vi "reward_behavior_michelle_visjitter_conswinAdapt_enticefx_TSLog_VF.vi"() -> ()   [LabVIEW 2019]
doc: "The myRIO Project template acquires acceleration data from the onboard accelerometer and displays the changes of acceleration values in a waveform chart."
uses:
  <vilib>/Analysis/Matrix/Datatypes/RealMatrix.ctl
  <vilib>/myRIO/Instrument Drivers/Onboard IO/DIO/typedefs/DIO Reference.ctl
  <vilib>/myRIO/Common/Instrument Driver Framework/Utilities/typedefs/myRIO Generic Hardware Reference.ctl
  <vilib>/myRIO/Common/Instrument Driver Framework/Utilities/typedefs/Hardware Version Enum.ctl
  <vilib>/myRIO/Common/Instrument Driver Framework/Utilities/typedefs/myRIO v1.0 Reference.ctl
  <vilib>/myRIO/Common/Instrument Driver Framework/Utilities/typedefs/Generic FPGA Reference.ctl
  <vilib>/myRIO/Common/Instrument Driver Framework/myRIO v1.0/DIO/typedefs/DIO Channels List.ctl
  <vilib>/myRIO/Common/Instrument Driver Framework/myRIO v1.0/DIO/typedefs/DIO Channels Enum.ctl
  <vilib>/userdefined/High Color/nirio_resource_hc.ctl
  <vilib>/myRIO/Common/Instrument Driver Framework/myRIO v1.0/Encoder/typedefs/Encoder Signal Mode.ctl
  <vilib>/myRIO/Instrument Drivers/Onboard IO/Encoder/typedefs/Encoder Reference.ctl
  <vilib>/myRIO/Common/Instrument Driver Framework/myRIO v1.0/Encoder/typedefs/Encoder Channels Enum.ctl
  <vilib>/myRIO/Common/Instrument Driver Framework/myRIO v1.0/Encoder/typedefs/Encoder Configuration v1.0.ctl
  <vilib>/myRIO/Common/Instrument Driver Framework/Utilities/vis/Is FPGA Ref Available.vi
  <vilib>/myRIO/Common/Instrument Driver Framework/myRIO v1.0/DIO/vis/myRIO v1.1 Open DIO.vi
  <vilib>/myRIO/Instrument Drivers/Onboard IO/DIO/vis/Write.vi
  <vilib>/myRIO/Common/Instrument Driver Framework/myRIO v1.0/Encoder/vis/myRIO v1.1 Open Encoder.vi
  <vilib>/myRIO/Instrument Drivers/Onboard IO/Encoder/vis/Read.vi
  <vilib>/myRIO/Instrument Drivers/Onboard IO/DIO/vis/Read.vi
  <vilib>/myRIO/Common/Instrument Driver Framework/Utilities/vis/Validate Channels.vi
  <vilib>/myRIO/Common/Instrument Driver Framework/myRIO v1.0/DIO/vis/myRIO v1.0 Reserve DIO.vi
  <vilib>/myRIO/Common/Instrument Driver Framework/myRIO v1.0/Encoder/vis/myRIO v1.0 Reserve Encoder.vi
  <vilib>/myRIO/Common/Instrument Driver Framework/myRIO v1.0/Resource Manager/vis/myRIO v1.0 Reserve Channel List.vi
  <vilib>/myRIO/Common/Instrument Driver Framework/myRIO v1.0/DIO/vis/myRIO v1.0 Build MUX Configuration DIO.vi
  <vilib>/myRIO/Common/Instrument Driver Framework/myRIO v1.0/Encoder/vis/myRIO v1.0 Build MUX Configuration Encoder.vi
  <vilib>/myRIO/Common/Instrument Driver Framework/myRIO v1.0/Resource Manager/vis/myRIO v1.0 Reserve Channel.vi
  <vilib>/myRIO/Common/Instrument Driver Framework/myRIO v1.0/Resource Manager/vis/myRIO v1.0 Unreserve Channel.vi
  <vilib>/myRIO/Common/Instrument Driver Framework/myRIO v1.0/Resource Manager/vis/myRIO v1.0 Create Configuration List.vi
  <vilib>/myRIO/Common/Instrument Driver Framework/myRIO v1.0/Resource Manager/vis/myRIO v1.0 Build Mutex Name.vi
  <vilib>/Utility/VariantDataType/GetNumericInfo.vi
  <vilib>/Utility/error.llb/Error Cluster From Error Code.vi
  <vilib>/myRIO/Common/Instrument Driver Framework/myRIO v1.0/myRIO v1.1 Open.vi
  <vilib>/myRIO/Common/Instrument Driver Framework/Utilities/vis/IO Manager.vi
  <vilib>/myRIO/Common/Instrument Driver Framework/Utilities/vis/Configuration Manager.vi
  <vilib>/myRIO/Common/Instrument Driver Framework/myRIO v1.0/Resource Manager/vis/myRIO v1.0 Configure IO.vi
  <vilib>/myRIO/Common/Instrument Driver Framework/myRIO v1.0/myRIO v1.0 Close.vi
  <vilib>/myRIO/Common/Instrument Driver Framework/myRIO v1.0/Encoder/vis/myRIO v1.0 Configure Encoder.vi
  <vilib>/myRIO/Common/Instrument Driver Framework/myRIO v1.0/Encoder/vis/myRIO v1.0 Read Encoder.vi
  <vilib>/myRIO/Common/Instrument Driver Framework/myRIO v1.0/DIO/vis/myRIO v1.0 Write DIO.vi
  <vilib>/myRIO/Common/Instrument Driver Framework/myRIO v1.0/DIO/vis/myRIO v1.0 Read DIO.vi
  <vilib>/myRIO/Express VI/Onboard IO/Encoder/Encoder Express VI.xnode
  <vilib>/myRIO/Instrument Drivers/Onboard IO/Encoder/vis/myRIO Encoder Open.xnode
  <vilib>/myRIO/Common/Instrument Driver Framework/myRIO v1.0/Encoder/typedefs/Encoder Count Direction Enum.ctl
  <vilib>/myRIO/Express VI/Onboard IO/DO/DO Express VI.xnode
  <vilib>/myRIO/Instrument Drivers/Onboard IO/DIO/vis/myRIO DIO Open.xnode
  <vilib>/myRIO/Express VI/Onboard IO/DI/DI Express VI.xnode
  <vilib>/myRIO/Instrument Drivers/Onboard IO/Encoder/Encoder.lvlib
  <vilib>/myRIO/Instrument Drivers/Onboard IO/DIO/DIO.lvlib
  <vilib>/Analysis/Matrix/NI_Matrix.lvlib
panel:
  out "AutoEnticeLimit":i32=1000
  out "GetVidFrame":i32
  out "VidTS":dbl[][](array[numeric])
  out "VidFrameClock":i32
  out "EntTS":dbl[][](array[numeric])
  out "TimeLag":dbl
  out "Lag2":dbl
  out "TestTime":dbl
  out "RewTS":dbl[][](array[numeric])
  out "ConsTS":dbl[][](array[numeric])
  out "LickTS":dbl[][](array[numeric])
  out "ContrastChoice":dbl
  out "Its":i32
  out "BurstCriteria":dbl
  out "LickBurst 2":bool
  out "LickBurst":bool
  out "Enticements":i32
  in  "Entice":bool
  out "Misses":i32
  out "GoAhead":bool
  out "TimeOutDuration":i32
  out "ActiveTime":dbl
  out "ConsumptionGo":bool=TRUE
  out "Consumption_Period":i32
  out "Watch_Display":bool=TRUE
  in  "Give reward":bool
  out "Timings":dbl[](array[numeric])
  out "ISI":dbl
  out "ISI start time":dbl
  out "Time_out":bool=TRUE
  out "Time since lick":dbl
  out "Time of last lick":dbl
  out "Rewarded trials":dbl[](array[numeric])
  out "Rewards":u16
  out "Active Trial":bool
  out "Array temp2":T1
  out "Stimuli Loaded":bool
  out "Stim_ID":dbl[](array[numeric])
  out "Reward_mat":dbl[](array[numeric])
  out "Reward":bool=TRUE
  out "Frame clock":i32
  out "Licks":u32
  out "Lick":bool
  out "Time":dbl
  out "Stop":bool
  in  "Frames to collect":u32
  out "Overflow?":bool
  out "Counter Value":i32
  out "Velocity":dbl
  out "Velocity Plot":dbl[](graph)
  out "Velocity array":dbl[](array[numeric])
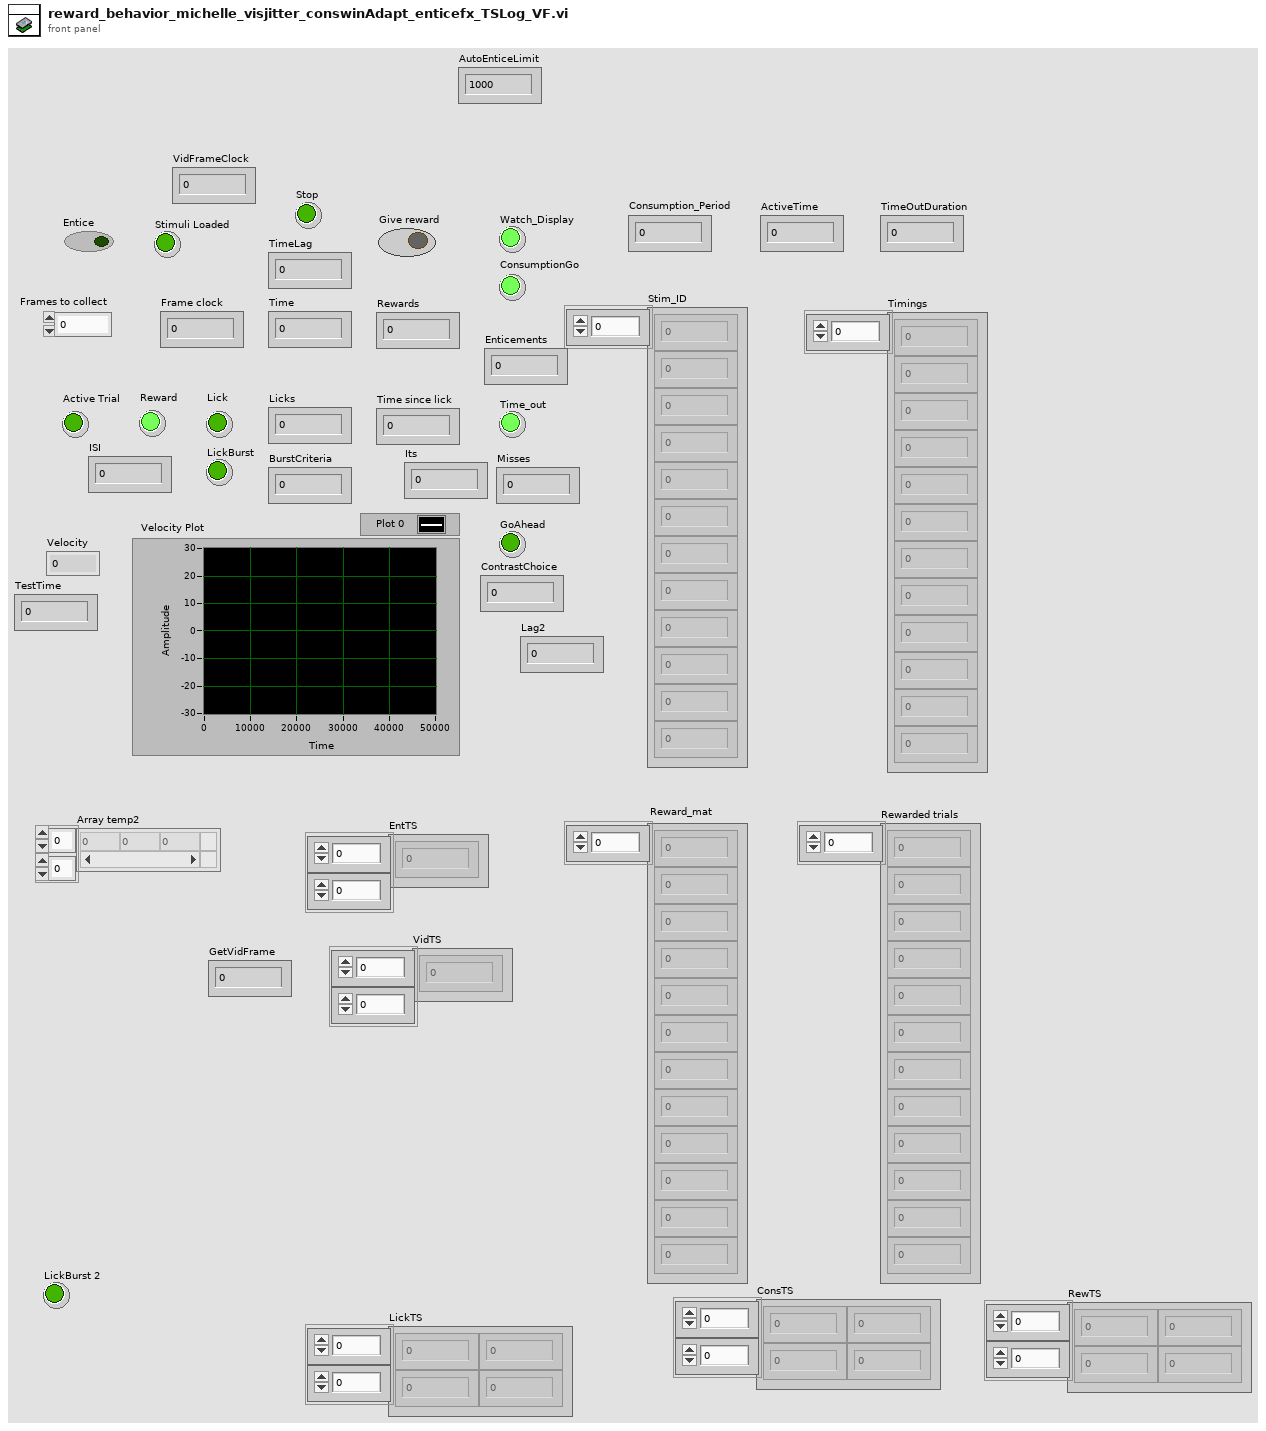
[diagram p1: front panel]
types:
  T1 = typedef "NI_Matrix.lvlib/RealMatrix.ctl" = dbl[][]
  T2 = typedef "DIO.lvlib/DIO Reference.ctl" = cluster{"myRIO Reference":T3, "DIO Channels List":T7}
  T3 = typedef "myRIO Generic Hardware Reference.ctl" = cluster{"myRIO Model":T4, "myRIO Hardware Reference":T5}
  T4 = typedef "Hardware Version Enum.ctl" = enum16{"Unknown", "myRIO-1900", "myRIO-1950", "roboRIO", "NI ELVIS RIO CM", "ELVIS III"}
  T5 = typedef "myRIO v1.0 Reference.ctl" = cluster{"Generic FPGA Reference":T6, "Allow multiple opens":bool}
  T6 = typedef "Generic FPGA Reference.ctl" = refnum<k20>
  T7 = typedef "DIO Channels List.ctl" = T8[]
  T8 = typedef "DIO Channels Enum.ctl" = enum16{"Not Connected", "C/DIO0", "C/DIO1", "C/DIO2", "C/DIO3", "C/DIO4", "C/DIO5", "C/DIO6", "C/DIO7", "A/DIO0", "A/DIO1", "A/DIO2", "A/DIO3", "A/DIO4", "A/DIO5", "A/DIO6", "A/DIO7", "A/DIO8", "A/DIO9", "A/DIO10", "A/DIO11", "A/DIO12", "A/DIO13", "A/DIO14", "A/DIO15", "A/DIO16", "A/DIO17", "A/DIO18", "A/DIO19", "B/DIO0", "B/DIO1", "B/DIO2", "B/DIO3", "B/DIO4", "B/DIO5", "B/DIO6", "B/DIO7", "B/DIO8", "B/DIO9", "B/DIO10", "B/DIO11", "B/DIO12", "B/DIO13", "B/DIO14", "B/DIO15", "B/DIO16", "B/DIO17", "B/DIO18", "B/DIO19", "LED0", "LED1", "LED2", "LED3", "Button0", "DIO/DIO0", "DIO/DIO1", "DIO/DIO2", "DIO/DIO3", "DIO/DIO4", "DIO/DIO5", "DIO/DIO6", "DIO/DIO7", "DIO/DIO8", "DIO/DIO9", "SPI/CS0", "SPI/CS1", "SPI/CS2", "SPI/CS3", "LED RADIO (Green)", "LED RADIO (Red)", "LED COMM (Green)", "LED COMM (Red)", "LED MODE (Green)", "LED MODE (Red)"}
  T9 = typedef "nirio_resource_hc.ctl" = tag
  T10 = typedef "Encoder.lvlib/Encoder Reference.ctl" = cluster{"myRIO Reference":T3, "Encoder Channels Enum":T11}
  T11 = typedef "Encoder Channels Enum.ctl" = enum16{"Not Connected", "C/ENC0", "C/ENC1", "A/ENC", "A/ENC0", "A/ENC1", "A/ENC2", "A/ENC3", "A/ENC4", "A/ENC5", "A/ENC6", "A/ENC7", "A/ENC8", "A/ENC9", "B/ENC", "B/ENC0", "B/ENC1", "B/ENC2", "B/ENC3", "B/ENC4", "B/ENC5", "B/ENC6", "B/ENC7", "B/ENC8", "B/ENC9", "DIO/ENC0", "DIO/ENC1", "DIO/ENC2", "DIO/ENC3", "DIO/ENC4"}
  T12 = typedef "Encoder Signal Mode.ctl" = enum16{"Quadrature phase signal", "Step and direction signal"}
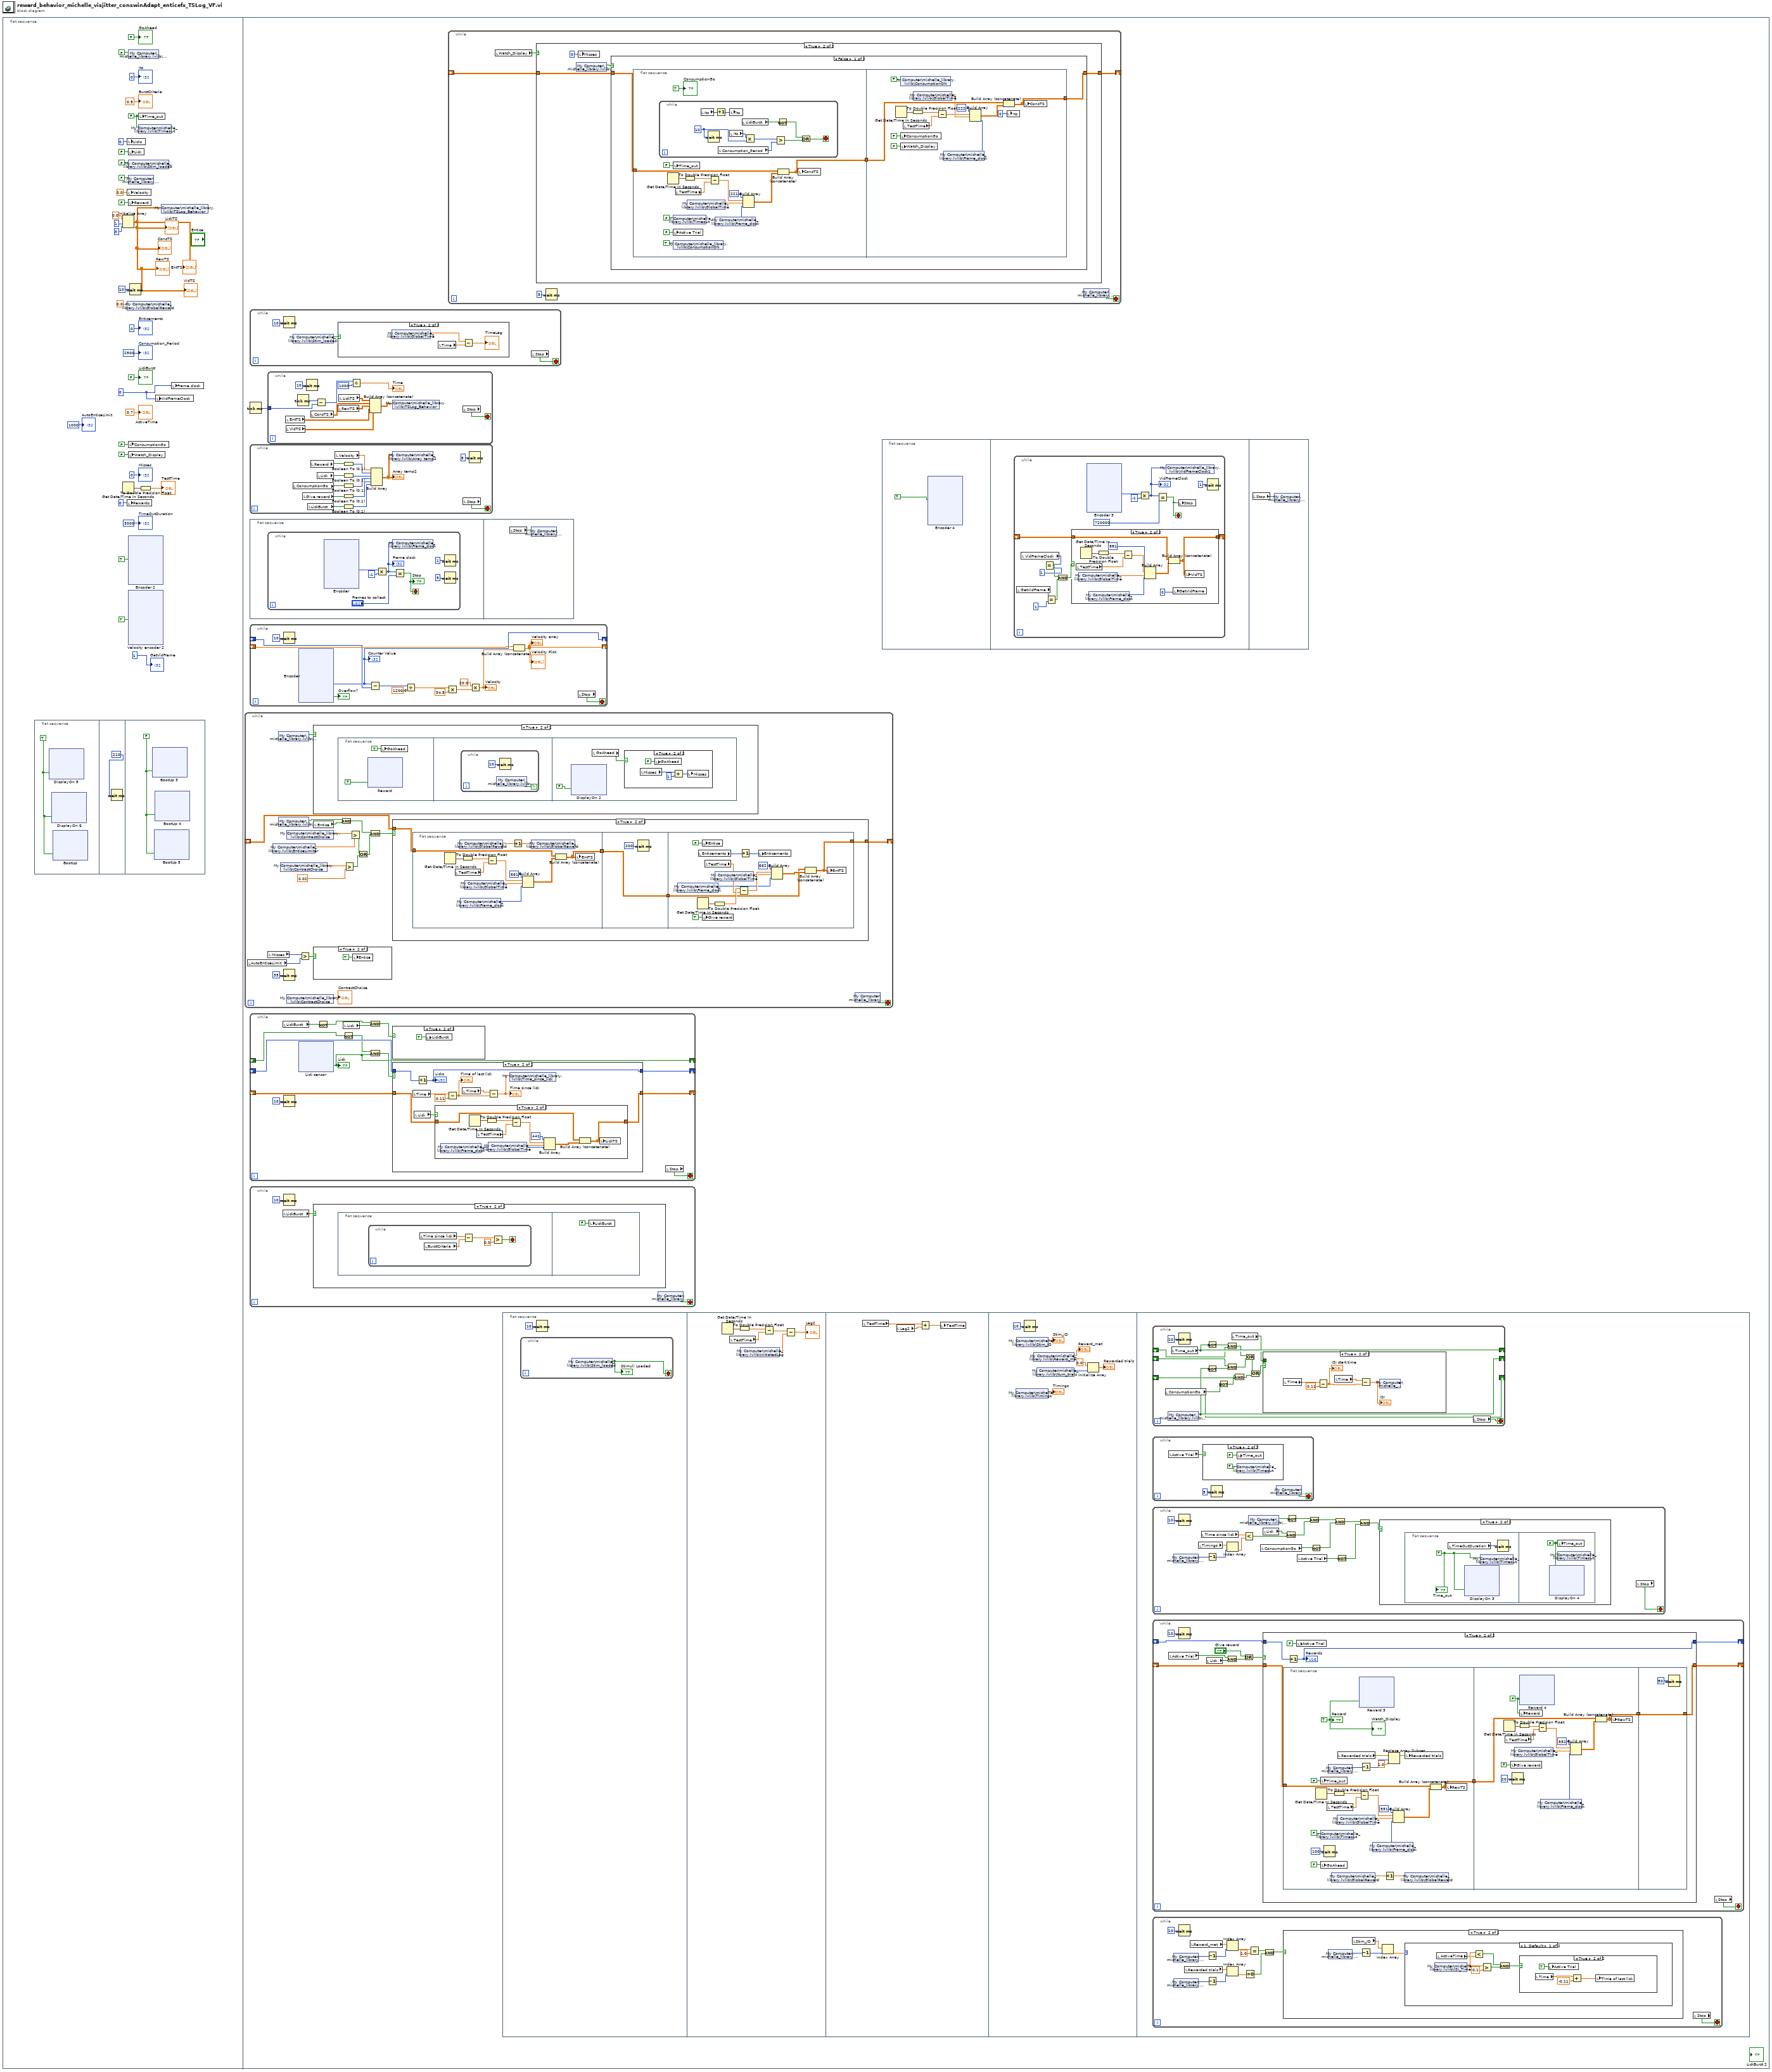
[diagram p0: block diagram]
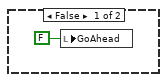
[diagram p7: hidden frame]
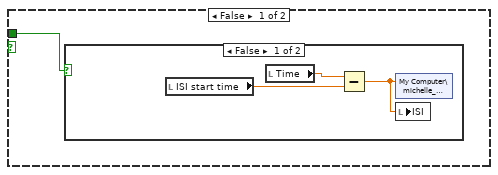
[diagram p13: hidden frame]
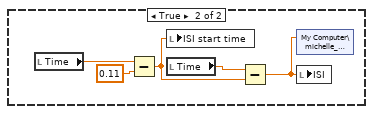
[diagram p14: hidden frame]
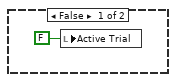
[diagram p15: hidden frame]
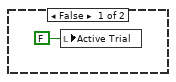
[diagram p16: hidden frame]
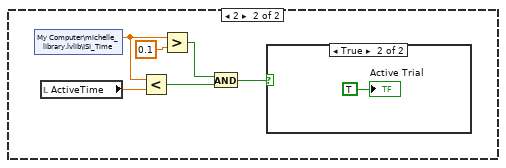
[diagram p17: hidden frame]
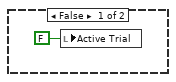
[diagram p18: hidden frame]
diagram:
  n1 = flat-sequence {
    frame #0 {
      w22 = FALSE ("Time_out")
      w4 = u32 0 ("Frames")
      n2 = flat-sequence {
        frame #0 {
          w34 = TRUE
          n3 = xnode "DisplayOn 5"("C/DIO2 (DIO2)"=w34) -> ()  [unwired: 1 in, 1 out]
          n4 = xnode "DisplayOn 6"("C/DIO1 (DIO1)"=w34) -> ()  [unwired: 1 in, 1 out]
          n5 = xnode "BootUp"("C/DIO3 (DIO3)"=w34) -> ()  [unwired: 1 in, 1 out]
        }
        frame #1 {
          n6 = Wait (ms)(milliseconds to wait=210) -> ()  [unwired: 1 out]
        }
        frame #2 {
          w141 = FALSE
          n7 = xnode "BootUp 3"("C/DIO2 (DIO2)"=w141) -> ()  [unwired: 1 in, 1 out]
          n8 = xnode "BootUp 5"("C/DIO3 (DIO3)"=w141) -> ()  [unwired: 1 in, 1 out]
          n9 = xnode "BootUp 4"("C/DIO1 (DIO1)"=w141) -> ()  [unwired: 1 in, 1 out]
        }
      }
      n10 = Get Date/Time In Seconds() -> (seconds since 1Jan1904=w6:timestamp)
      n11 = Initialize Array(0.0, 1, 3) -> (w3:dbl[][])
      "LickTS" <- w3
      "ConsTS" <- w3
      "RewTS" <- w3
      "EntTS" <- w3
      "VidTS" <- w3
      n12 = local write "Licks"(u32 0 ("Licks")) -> ()
      n13 = local write "Velocity"(0.0 ("Velocity")) -> ()
      n14 = shared-variable "My Computer\\michelle_library.lvlib\\GlobalReward"(0.0) -> ()  [unwired: 1 in, 1 out]
      n15 = local write "Rewards"(u16 0 ("Rewards")) -> ()
      n16 = shared-variable "My Computer\\michelle_library.lvlib\\Display"(FALSE ("Display")) -> ()  [unwired: 1 in, 1 out]
      n17 = local write "Lick"(FALSE ("Lick")) -> ()
      n18 = shared-variable "My Computer\\michelle_library.lvlib\\Stim_loaded"(FALSE ("Stim_loaded")) -> ()  [unwired: 1 in, 1 out]
      n19 = shared-variable "My Computer\\michelle_library.lvlib\\Stop"(FALSE ("Stop")) -> ()  [unwired: 1 in, 1 out]
      n20 = local write "Reward"(FALSE ("Give reward")) -> ()
      n21 = local write "ConsumptionGo"(FALSE ("ConsumptionGo")) -> ()
      n22 = local write "Watch_Display"(FALSE ("Watch_Display")) -> ()
      n23 = xnode "Encoder 2"("Reset Counter"=TRUE) -> ()  [unwired: 1 in, 4 out]
      n24 = xnode "Velocity encoder 2"("Reset Counter"=TRUE) -> ()  [unwired: 1 in, 4 out]
      n25 = Wait (ms)(milliseconds to wait=u32 10) -> ()  [unwired: 1 out]
      n26 = local write "Time_out"(w22) -> ()
      n27 = shared-variable "My Computer\\michelle_library.lvlib\\Timeout"(w22) -> ()  [unwired: 1 in, 1 out]
      n28 = To Double Precision Float(number=w6) -> (double precision float=→"TestTime":dbl)
      n29 = local write "VidFrameClock"(w4) -> ()
      n30 = shared-variable "My Computer\\michelle_library.lvlib\\TSLog_Behavior"(w3) -> ()  [unwired: 1 in, 1 out]
      n31 = local write "Frame clock"(w4) -> ()
      "Consumption_Period" <- 2500
      "ActiveTime" <- 0.7
      "TimeOutDuration" <- 3000
      "GoAhead" <- FALSE
      "Misses" <- 0
      "Enticements" <- 0
      "LickBurst" <- FALSE
      "BurstCriteria" <- 0.5
      "Its" <- 0
      "GetVidFrame" <- 1
      "AutoEnticeLimit" <- 1000
    }
    frame #1 {
      n32 = while {
        shift-right: [w484] -> _
        shift-left: _ -> [w485]
        stop <- w495 stop-if-true
        n33 = local read "AutoEnticeLimit"() -> (w476:i32)
        n34 = local read "Misses"() -> (w477:i32)
        n35 = shared-variable "My Computer\\michelle_library.lvlib\\EnticeLimiter"() -> (w483:dbl)  [unwired: 1 in, 1 out]
        n36 = shared-variable "My Computer\\michelle_library.lvlib\\Display"() -> (w494:bool)  [unwired: 1 in, 1 out]
        n37 = shared-variable "My Computer\\michelle_library.lvlib\\Display"() -> (w492:bool)  [unwired: 1 in, 1 out]
        n38 = shared-variable "My Computer\\michelle_library.lvlib\\ContrastChoice"() -> (w479:dbl)  [unwired: 1 in, 1 out]
        n39 = Wait (ms)(milliseconds to wait=35) -> ()  [unwired: 1 out]
        n40 = shared-variable "My Computer\\michelle_library.lvlib\\ContrastChoice"() -> (w488:dbl)  [unwired: 1 in, 1 out]
        n41 = shared-variable "My Computer\\michelle_library.lvlib\\ContrastChoice"() -> (→"ContrastChoice":dbl)  [unwired: 1 in, 1 out]
        n42 = Greater?(x=w477, y=w476) -> (0:w493:bool)
        n43 = case shown="True" w494 {
          frame False {
            n44 = local write "GoAhead"(FALSE) -> ()
          }
          frame True {
            n45 = flat-sequence {
              frame #0 {
                n46 = xnode "Reward"("C/DIO2 (DIO2)"=TRUE) -> ()  [unwired: 1 in, 1 out]
                n47 = local write "GoAhead"(TRUE) -> ()
              }
              frame #1 {
                n48 = while {
                  stop <- w569 continue-if-true
                  n49 = shared-variable "My Computer\\michelle_library.lvlib\\Display"() -> (w569:bool)  [unwired: 1 in, 1 out]
                  n50 = Wait (ms)(milliseconds to wait=10) -> ()  [unwired: 1 out]
                }
              }
              frame #2 {
                n51 = xnode "DisplayOn 2"("C/DIO2 (DIO2)"=FALSE) -> ()  [unwired: 1 in, 1 out]
                n52 = local read "GoAhead"() -> (w571:bool)
                n53 = case shown="True" w571 {
                  frame False {
                  }
                  frame True {
                    n54 = local read "Misses"() -> (w610:i32)
                    n55 = local write "GoAhead"(FALSE) -> ()
                    n56 = Add(x=w610, y=1) -> (x+y=w608:i32)
                    n57 = local write "Misses"(w608) -> ()
                  }
                }
              }
            }
          }
        }
        n58 = local read "Entice"() -> (w491:bool)
        n59 = case shown="True" w493 {
          frame False {
          }
          frame True {
            n60 = local write "Entice"(TRUE) -> ()
          }
        }
        n61 = And(x=w492, y=w491) -> (x .and. y?=w489:bool)
        n62 = Greater?(x=w479, y=0.02) -> (0:w480:bool)
        n63 = Greater?(x=w488, y=w483) -> (0:w481:bool)
        n64 = Or(x=w481, y=w480) -> (x .or. y?=w482:bool)
        n65 = And(x=w489, y=w482) -> (x .and. y?=w487:bool)
        n66 = case shown="True" w487 {
          tunnel: w485 -> [w496 w500]
          tunnel: [w496 w497] -> w484
          frame False {
          }
          frame True {
            n67 = flat-sequence {
              tunnel: w500 -> [w503]
              tunnel: [w502] -> w499
              tunnel: w499 -> [w513]
              tunnel: [w513] -> w498
              tunnel: w498 -> [w517]
              tunnel: [w516] -> w497
              frame #0 {
                n68 = Get Date/Time In Seconds() -> (seconds since 1Jan1904=w510:timestamp)
                n69 = local read "TestTime"() -> (w505:dbl)
                n70 = shared-variable "My Computer\\michelle_library.lvlib\\GlobalReward"() -> (w512:dbl)  [unwired: 1 in, 1 out]
                n71 = shared-variable "My Computer\\michelle_library.lvlib\\Frame_clock"() -> (w501:u32)  [unwired: 1 in, 1 out]
                n72 = To Double Precision Float(number=w510) -> (double precision float=w509:dbl)
                n73 = shared-variable "My Computer\\michelle_library.lvlib\\GlobalTime"() -> (w504:dbl)  [unwired: 1 in, 1 out]
                n74 = Subtract(x=w509, y=w505) -> (x-y=w508:dbl)
                n75 = Increment(x=w512) -> (x+1=w511:dbl)
                n76 = Build Array(661, w508, w504, w501) -> (w507:T1)
                n77 = shared-variable "My Computer\\michelle_library.lvlib\\GlobalReward"(w511) -> ()  [unwired: 1 in, 1 out]
                n78 = Build Array (concatenate) ("Build Matrix")(w503, w507) -> (w502:T1)
                n79 = local write "EntTS"(w502) -> ()
              }
              frame #1 {
                n80 = Wait (ms)(milliseconds to wait=200) -> ()  [unwired: 1 out]
              }
              frame #2 {
                n81 = shared-variable "My Computer\\michelle_library.lvlib\\Frame_clock"() -> (w515:u32)  [unwired: 1 in, 1 out]
                n82 = Get Date/Time In Seconds() -> (seconds since 1Jan1904=w524:timestamp)
                n83 = local read "Enticements"() -> (w526:i32)
                n84 = local write "Entice"(FALSE) -> ()
                n85 = local write "Give reward"(TRUE) -> ()
                n86 = local read "TestTime"() -> (w518:dbl)
                n87 = To Double Precision Float(number=w524) -> (double precision float=w523:dbl)
                n88 = shared-variable "My Computer\\michelle_library.lvlib\\GlobalTime"() -> (w519:dbl)  [unwired: 1 in, 1 out]
                n89 = Subtract(x=w523, y=w518) -> (x-y=w522:dbl)
                n90 = Increment(x=w526) -> (x+1=w525:i32)
                n91 = local write "Enticements"(w525) -> ()
                n92 = Build Array(662, w522, w519, w515) -> (w521:T1)
                n93 = Build Array (concatenate) ("Build Matrix")(w517, w521) -> (w516:T1)
                n94 = local write "EntTS"(w516) -> ()
              }
            }
          }
        }
        n95 = shared-variable "My Computer\\michelle_library.lvlib\\Stop"() -> (w495:bool)  [unwired: 1 in, 1 out]
      }
      n96 = while {
        stop <- w462 stop-if-true
        n97 = Wait (ms)(milliseconds to wait=u32 10) -> ()  [unwired: 1 out]
        n98 = shared-variable "My Computer\\michelle_library.lvlib\\Stim_loaded"() -> (w463:bool)  [unwired: 1 in, 1 out]
        n99 = case shown="True" w463 {
          frame False {
          }
          frame True {
            n100 = shared-variable "My Computer\\michelle_library.lvlib\\GlobalTime"() -> (w464:dbl)  [unwired: 1 in, 1 out]
            n101 = local read "Time"() -> (w465:dbl)
            n102 = Subtract(x=w464, y=w465) -> (x-y=→"TimeLag":dbl)
          }
        }
        n103 = local read "Stop"() -> (w462:bool)
      }
      n104 = Tick Count (ms)() -> (millisecond timer value=w339:u32)
      n105 = while {
        stop <- w671 stop-if-true
        n106 = local read "ConsumptionGo"() -> (w669:bool)
        n107 = local read "Give reward"() -> (w668:bool)
        n108 = local read "LickBurst"() -> (w665:bool)
        n109 = local read "Reward"() -> (w676:bool)
        n110 = local read "Lick"() -> (w677:bool)
        n111 = local read "Velocity"() -> (w675:dbl)
        n112 = Boolean To (0,1)(Boolean=w676) -> (0, 1=w674:i16)
        n113 = Boolean To (0,1)(Boolean=w677) -> (0, 1=w673:i16)
        n114 = Boolean To (0,1)(Boolean=w669) -> (0, 1=w667:i16)
        n115 = Boolean To (0,1)(Boolean=w668) -> (0, 1=w666:i16)
        n116 = Boolean To (0,1)(Boolean=w665) -> (0, 1=w664:i16)
        n117 = Build Array(w675, w674, w673, w667, w666, w664) -> (w670:T1)
        "Array temp2" <- w670
        n118 = shared-variable "My Computer\\michelle_library.lvlib\\Array temp2"(w670) -> ()  [unwired: 1 in, 1 out]
        n119 = local read "Stop"() -> (w671:bool)
        n120 = Wait (ms)(milliseconds to wait=u32 5) -> ()  [unwired: 1 out]
      }
      n121 = flat-sequence {
        frame #0 {
          n122 = while {
            stop <- w990 stop-if-true
            n123 = xnode "Encoder"() -> ("Counter Value"=w994:i32)  [unwired: 2 in, 3 out]
            n124 = Multiply(x=w994, y=-1) -> (x*y=w989:i32)
            "Frame clock" <- w989
            n125 = shared-variable "My Computer\\michelle_library.lvlib\\Frame_clock"(w989) -> ()  [unwired: 1 in, 1 out]
            n126 = Equal?(x=w989, y="Frames to collect") -> (x = y?=w990:bool)
            "Stop" <- w990
            n127 = Wait (ms)(milliseconds to wait=u32 1) -> ()  [unwired: 1 out]
            n128 = Wait (ms)(milliseconds to wait=u32 5) -> ()  [unwired: 1 out]
          }
        }
        frame #1 {
          n129 = local read "Stop"() -> (w1042:bool)
          n130 = shared-variable "My Computer\\michelle_library.lvlib\\Stop"(w1042) -> ()  [unwired: 1 in, 1 out]
        }
      }
      n131 = while {
        shift-right: [w1129] -> _
        shift-left: _ -> [w1130]
        shift-right: [w1121] -> _
        shift-left: _ -> [w1120]
        stop <- w1119 stop-if-true
        n132 = Wait (ms)(milliseconds to wait=u32 10) -> ()  [unwired: 1 out]
        n133 = xnode "Encoder"() -> ("Counter Value"=w1129:i32, "Overflow?"=→"Overflow?":bool)  [unwired: 2 in, 2 out]
        "Counter Value" <- w1129
        n134 = Subtract(x=w1129, y=w1130) -> (x-y=w1122:i32)
        n135 = Divide(x=w1122, y=1200.0 ("600")) -> (x/y=w1127:dbl)
        n136 = Multiply(x=w1127, y=34.5) -> (x*y=w1125:dbl)
        n137 = Multiply(x=20.0, y=w1125) -> (x*y=w1123:dbl)
        "Velocity" <- w1123
        n138 = Build Array (concatenate)(w1120, w1123) -> (w1121:dbl[])
        "Velocity Plot" <- w1121
        "Velocity array" <- w1121
        n139 = local read "Stop"() -> (w1119:bool)
      }
      n140 = while {
        shift-right: [w1055] -> _
        shift-left: _ -> [w1054]
        shift-right: [w1049] -> _
        shift-left: _ -> [w1052]
        shift-right: [w1043] -> _
        shift-left: _ -> [w1044]
        stop <- w1053 stop-if-true
        n141 = local read "LickBurst"() -> (w1046:bool)
        n142 = Wait (ms)(milliseconds to wait=u32 10) -> ()  [unwired: 1 out]
        n143 = xnode "Lick sensor"() -> ("C/DIO1 (DIO1)"=w1049:bool)  [unwired: 1 in, 1 out]
        "Lick" <- w1049
        n144 = Not(x=w1046) -> (.not. x?=w1045:bool)
        n145 = Not(x=w1052) -> (.not. x?=w1051:bool)
        n146 = local read "Lick"() -> (w1047:bool)
        n147 = And(x=w1045, y=w1047) -> (x .and. y?=w1048:bool)
        n148 = And(x=w1051, y=w1049) -> (x .and. y?=w1050:bool)
        n149 = case shown="True" w1048 {
          frame False {
          }
          frame True {
            n150 = local write "LickBurst"(TRUE) -> ()
          }
        }
        n151 = case shown="True" w1050 {
          tunnel: [w1062 w1072] -> w1055
          tunnel: w1054 -> [w1062 w1071]
          tunnel: w1044 -> [w1058 w1063]
          tunnel: [w1058 w1065] -> w1043
          frame False {
            n152 = local read "Time of last lick"() -> (w1060:dbl)
            n153 = local read "Time"() -> (w1061:dbl)
            n154 = Subtract(x=w1061, y=w1060) -> (x-y=w1059:dbl)
            n155 = shared-variable "My Computer\\michelle_library.lvlib\\Time_since_lick"(w1059) -> ()  [unwired: 1 in, 1 out]
            n156 = local write "Time since lick"(w1059) -> ()
          }
          frame True {
            n157 = local read "Time"() -> (w1068:dbl)
            n158 = local read "Lick"() -> (w1064:bool)
            n159 = Increment(x=w1071) -> (x+1=w1072:u32)
            "Licks" <- w1072
            n160 = case shown="True" w1064 {
              tunnel: w1063 -> [w1073 w1079]
              tunnel: [w1073 w1078] -> w1065
              frame False {
              }
              frame True {
                n161 = shared-variable "My Computer\\michelle_library.lvlib\\Frame_clock"() -> (w1074:u32)  [unwired: 1 in, 1 out]
                n162 = Get Date/Time In Seconds() -> (seconds since 1Jan1904=w1081:timestamp)
                n163 = local read "TestTime"() -> (w1076:dbl)
                n164 = To Double Precision Float(number=w1081) -> (double precision float=w1077:dbl)
                n165 = shared-variable "My Computer\\michelle_library.lvlib\\GlobalTime"() -> (w1075:dbl)  [unwired: 1 in, 1 out]
                n166 = Subtract(x=w1077, y=w1076) -> (x-y=w1082:dbl)
                n167 = Build Array(441, w1082, w1075, w1074) -> (w1083:T1)
                n168 = Build Array (concatenate) ("Build Matrix")(w1079, w1083) -> (w1078:T1)
                n169 = local write "LickTS"(w1078) -> ()
              }
            }
            n170 = Subtract(x=w1068, y=0.11) -> (x-y=w1066:dbl)
            "Time of last lick" <- w1066
            n171 = local read "Time"() -> (w1070:dbl)
            n172 = Subtract(x=w1070, y=w1066) -> (x-y=w1069:dbl)
            "Time since lick" <- w1069
            n173 = shared-variable "My Computer\\michelle_library.lvlib\\Time_since_lick"(w1069) -> ()  [unwired: 1 in, 1 out]
          }
        }
        n174 = local read "Stop"() -> (w1053:bool)
      }
      n175 = while {
        stop <- w469 stop-if-true
        n176 = local read "LickBurst"() -> (w467:bool)
        n177 = Wait (ms)(milliseconds to wait=u32 10) -> ()  [unwired: 1 out]
        n178 = case shown="True" w467 {
          frame False {
          }
          frame True {
            n179 = flat-sequence {
              frame #0 {
                n180 = while {
                  stop <- w472 stop-if-true
                  n181 = local read "Time since lick"() -> (w473:dbl)
                  n182 = local read "BurstCriteria"() -> (w474:dbl)
                  n183 = Subtract(x=w473, y=w474) -> (x-y=w470:dbl)
                  n184 = Greater?(x=w470, y=0.0) -> (0:w472:bool)
                }
              }
              frame #1 {
                n185 = local write "LickBurst"(FALSE) -> ()
              }
            }
          }
        }
        n186 = shared-variable "My Computer\\michelle_library.lvlib\\Stop"() -> (w469:bool)  [unwired: 1 in, 1 out]
      }
      n187 = while {
        tunnel: w339 -> [w1190]
        stop <- w1188 stop-if-true
        n188 = local read "EntTS"() -> (w1180:dbl[][])
        n189 = local read "VidTS"() -> (w1179:dbl[][])
        n190 = Tick Count (ms)() -> (millisecond timer value=w1191:u32)
        n191 = Wait (ms)(milliseconds to wait=u32 10) -> ()  [unwired: 1 out]
        n192 = local read "ConsTS"() -> (w1183:dbl[][])
        n193 = Subtract(x=w1191, y=w1190) -> (x-y=w1187:u32)
        n194 = local read "RewTS"() -> (w1182:dbl[][])
        n195 = local read "LickTS"() -> (w1184:dbl[][])
        n196 = Divide(x=w1187, y=u32 1000) -> (x/y=→"Time":dbl)
        n197 = Build Array (concatenate) ("Build Matrix")(w1184, w1183, w1182, w1180, w1179) -> (w1181:T1)
        n198 = shared-variable "My Computer\\michelle_library.lvlib\\TSLog_Behavior"(w1181) -> ()  [unwired: 1 in, 1 out]
        n199 = local read "Stop"() -> (w1188:bool)
      }
      n200 = while {
        shift-right: [w611] -> _
        shift-left: _ -> [w612]
        stop <- w615 stop-if-true
        n201 = local read "Watch_Display"() -> (w614:bool)
        n202 = case shown="True" w614 {
          tunnel: w612 -> [w616 w618]
          tunnel: [w616 w617] -> w611
          frame False {
          }
          frame True {
            n203 = shared-variable "My Computer\\michelle_library.lvlib\\Display"() -> (w620:bool)  [unwired: 1 in, 1 out]
            n204 = local write "Misses"(0) -> ()
            n205 = case shown="False" w620 {
              tunnel: w618 -> [w623 w663]
              tunnel: [w621 w663] -> w617
              frame False {
                n206 = flat-sequence {
                  tunnel: w623 -> [w627]
                  tunnel: [w626] -> w622
                  tunnel: w622 -> [w653]
                  tunnel: [w652] -> w621
                  frame #0 {
                    n207 = while {
                      stop <- w642 stop-if-true
                      w643 = 10
                      n208 = local read "Its"() -> (w647:i32)
                      n209 = Wait (ms)(milliseconds to wait=w643) -> ()  [unwired: 1 out]
                      n210 = Increment(x=w647) -> (x+1=w646:i32)
                      n211 = local read "Consumption_Period"() -> (w640:i32)
                      n212 = local write "Its"(w646) -> ()
                      n213 = local read "Its"() -> (w644:i32)
                      n214 = local read "LickBurst"() -> (w648:bool)
                      n215 = Multiply(x=w644, y=w643) -> (x*y=w641:i32)
                      n216 = Greater?(x=w641, y=w640) -> (0:w639:bool)
                      n217 = Not(x=w648) -> (.not. x?=w645:bool)
                      n218 = Or(x=w645, y=w639) -> (x .or. y?=w642:bool)
                    }
                    n219 = Get Date/Time In Seconds() -> (seconds since 1Jan1904=w632:timestamp)
                    n220 = local write "Time_out"(FALSE) -> ()
                    n221 = shared-variable "My Computer\\michelle_library.lvlib\\Timeout"(FALSE) -> ()  [unwired: 1 in, 1 out]
                    n222 = local write "Active Trial"(FALSE) -> ()
                    n223 = shared-variable "My Computer\\michelle_library.lvlib\\ConsumptionON"(TRUE) -> ()  [unwired: 1 in, 1 out]
                    n224 = local read "TestTime"() -> (w629:dbl)
                    n225 = To Double Precision Float(number=w632) -> (double precision float=w630:dbl)
                    n226 = shared-variable "My Computer\\michelle_library.lvlib\\GlobalTime"() -> (w625:dbl)  [unwired: 1 in, 1 out]
                    n227 = Subtract(x=w630, y=w629) -> (x-y=w633:dbl)
                    n228 = shared-variable "My Computer\\michelle_library.lvlib\\Frame_clock"() -> (w624:u32)  [unwired: 1 in, 1 out]
                    n229 = Build Array(221, w633, w625, w624) -> (w628:T1)
                    n230 = Build Array (concatenate) ("Build Matrix")(w627, w628) -> (w626:T1)
                    n231 = local write "ConsTS"(w626) -> ()
                    "ConsumptionGo" <- TRUE
                  }
                  frame #1 {
                    n232 = Get Date/Time In Seconds() -> (seconds since 1Jan1904=w657:timestamp)
                    n233 = shared-variable "My Computer\\michelle_library.lvlib\\ConsumptionON"(FALSE) -> ()  [unwired: 1 in, 1 out]
                    n234 = local write "ConsumptionGo"(FALSE ("ConsumptionGo")) -> ()
                    n235 = local write "Watch_Display"(FALSE ("Watch_Display")) -> ()
                    n236 = local read "TestTime"() -> (w654:dbl)
                    n237 = To Double Precision Float(number=w657) -> (double precision float=w655:dbl)
                    n238 = shared-variable "My Computer\\michelle_library.lvlib\\GlobalTime"() -> (w650:dbl)  [unwired: 1 in, 1 out]
                    n239 = Subtract(x=w655, y=w654) -> (x-y=w658:dbl)
                    n240 = shared-variable "My Computer\\michelle_library.lvlib\\Frame_clock"() -> (w649:u32)  [unwired: 1 in, 1 out]
                    n241 = Build Array(222, w658, w650, w649) -> (w651:T1)
                    n242 = Build Array (concatenate) ("Build Matrix")(w653, w651) -> (w652:T1)
                    n243 = local write "Its"(0) -> ()
                    n244 = local write "ConsTS"(w652) -> ()
                  }
                }
              }
              frame True {
              }
            }
          }
        }
        n245 = Wait (ms)(milliseconds to wait=u32 5) -> ()  [unwired: 1 out]
        n246 = shared-variable "My Computer\\michelle_library.lvlib\\Stop"() -> (w615:bool)  [unwired: 1 in, 1 out]
      }
      n247 = flat-sequence {
        frame #0 {
          n248 = while {
            stop <- w679 stop-if-true
            n249 = shared-variable "My Computer\\michelle_library.lvlib\\Stim_loaded"() -> (w679:bool)  [unwired: 1 in, 1 out]
            "Stimuli Loaded" <- w679
          }
          n250 = Wait (ms)(milliseconds to wait=u32 10) -> ()  [unwired: 1 out]
        }
        frame #1 {
          n251 = Get Date/Time In Seconds() -> (seconds since 1Jan1904=w685:timestamp)
          n252 = local read "TestTime"() -> (w684:dbl)
          n253 = To Double Precision Float(number=w685) -> (double precision float=w683:dbl)
          n254 = shared-variable "My Computer\\michelle_library.lvlib\\InitiatedLag"() -> (w682:dbl)  [unwired: 1 in, 1 out]
          n255 = Subtract(x=w683, y=w684) -> (x-y=w680:dbl)
          n256 = Subtract(x=w680, y=w682) -> (x-y=→"Lag2":dbl)
        }
        frame #2 {
          n257 = local read "TestTime"() -> (w686:dbl)
          n258 = local read "Lag2"() -> (w687:dbl)
          n259 = Add(x=w686, y=w687) -> (x+y=w688:dbl)
          n260 = local write "TestTime"(w688) -> ()
        }
        frame #3 {
          n261 = shared-variable "My Computer\\michelle_library.lvlib\\Timings"() -> (→"Timings":dbl[])  [unwired: 1 in, 1 out]
          n262 = shared-variable "My Computer\\michelle_library.lvlib\\Stim_ID"() -> (→"Stim_ID":dbl[])  [unwired: 1 in, 1 out]
          n263 = Wait (ms)(milliseconds to wait=u32 10) -> ()  [unwired: 1 out]
          n264 = shared-variable "My Computer\\michelle_library.lvlib\\Reward_mat"() -> (→"Reward_mat":dbl[])  [unwired: 1 in, 1 out]
          n265 = shared-variable "My Computer\\michelle_library.lvlib\\Num_trials"() -> (w692:u32)  [unwired: 1 in, 1 out]
          n266 = Initialize Array(0.0 ("element"), w692) -> (→"Rewarded trials":dbl[])
        }
        frame #4 {
          n267 = while {
            shift-right: [w808] -> _
            shift-left: _ -> [w806]
            shift-right: [w804] -> _
            shift-left: _ -> [w803]
            shift-right: [w798] -> _
            shift-left: _ -> [w796]
            stop <- w809 stop-if-true
            n268 = local read "ConsumptionGo"() -> (w798:bool)
            n269 = shared-variable "My Computer\\michelle_library.lvlib\\Display"() -> (w804:bool)  [unwired: 1 in, 1 out]
            n270 = local read "Time_out"() -> (w808:bool)
            n271 = Wait (ms)(milliseconds to wait=u32 10) -> ()  [unwired: 1 out]
            n272 = Not(x=w808) -> (.not. x?=w807:bool)
            n273 = Not(x=w804) -> (.not. x?=w802:bool)
            n274 = Not(x=w798) -> (.not. x?=w799:bool)
            n275 = And(x=w807, y=w806) -> (x .and. y?=w801:bool)
            n276 = And(x=w803, y=w802) -> (x .and. y?=w797:bool)
            n277 = local read "Time_out"() -> (w805:bool)
            n278 = And(x=w796, y=w799) -> (x .and. y?=w795:bool)
            n279 = Or(x=w801, y=w797) -> (x .or. y?=w794:bool)
            n280 = Or(x=w794, y=w795) -> (x .or. y?=w793:bool)
            n281 = case shown="True" w793 {
              tunnel: w805 -> [w810 _]
              frame False {
                n282 = case shown="False" w810 {
                  frame False {
                    n283 = local read "ISI start time"() -> (w813:dbl)
                    n284 = local read "Time"() -> (w812:dbl)
                    n285 = Subtract(x=w812, y=w813) -> (x-y=w811:dbl)
                    n286 = shared-variable "My Computer\\michelle_library.lvlib\\ISI"(w811) -> ()  [unwired: 1 in, 1 out]
                    n287 = local write "ISI"(w811) -> ()
                  }
                  frame True {
                    n288 = local read "Time"() -> (w818:dbl)
                    n289 = Subtract(x=w818, y=0.11) -> (x-y=w815:dbl)
                    n290 = local write "ISI start time"(w815) -> ()
                    n291 = local read "Time"() -> (w816:dbl)
                    n292 = Subtract(x=w816, y=w815) -> (x-y=w814:dbl)
                    n293 = shared-variable "My Computer\\michelle_library.lvlib\\ISI"(w814) -> ()  [unwired: 1 in, 1 out]
                    n294 = local write "ISI"(w814) -> ()
                  }
                }
              }
              frame True {
                n295 = local read "Time"() -> (w823:dbl)
                n296 = Subtract(x=w823, y=0.11) -> (x-y=w820:dbl)
                "ISI start time" <- w820
                n297 = local read "Time"() -> (w821:dbl)
                n298 = Subtract(x=w821, y=w820) -> (x-y=w819:dbl)
                "ISI" <- w819
                n299 = shared-variable "My Computer\\michelle_library.lvlib\\ISI"(w819) -> ()  [unwired: 1 in, 1 out]
              }
            }
            n300 = local read "Stop"() -> (w809:bool)
          }
          n301 = while {
            stop <- w698 stop-if-true
            n302 = local read "Active Trial"() -> (w697:bool)
            n303 = case shown="True" w697 {
              frame False {
              }
              frame True {
                n304 = local write "Time_out"(FALSE) -> ()
                n305 = shared-variable "My Computer\\michelle_library.lvlib\\Timeout"(FALSE) -> ()  [unwired: 1 in, 1 out]
              }
            }
            n306 = Wait (ms)(milliseconds to wait=5) -> ()  [unwired: 1 out]
            n307 = shared-variable "My Computer\\michelle_library.lvlib\\Stop"() -> (w698:bool)  [unwired: 1 in, 1 out]
          }
          n308 = while {
            stop <- w719 stop-if-true
            n309 = shared-variable "My Computer\\michelle_library.lvlib\\Trial"() -> (w709:u32)  [unwired: 1 in, 1 out]
            n310 = Wait (ms)(milliseconds to wait=u32 10) -> ()  [unwired: 1 out]
            n311 = local read "Timings"() -> (w711:dbl[])
            n312 = local read "Time since lick"() -> (w718:dbl)
            n313 = Decrement(x=w709) -> (x-1=w708:u32)
            n314 = Index Array(array=w711, index=w708) -> (element=w710:dbl)
            n315 = Less?(x=w718, y=w710) -> (x < y?=w717:bool)
            n316 = shared-variable "My Computer\\michelle_library.lvlib\\Display"() -> (w714:bool)  [unwired: 1 in, 1 out]
            n317 = local read "ConsumptionGo"() -> (w706:bool)
            n318 = local read "Lick"() -> (w716:bool)
            n319 = And(x=w716, y=w717) -> (x .and. y?=w712:bool)
            n320 = Not(x=w714) -> (.not. x?=w713:bool)
            n321 = local read "Active Trial"() -> (w701:bool)
            n322 = And(x=w713, y=w712) -> (x .and. y?=w705:bool)
            n323 = Not(x=w706) -> (.not. x?=w707:bool)
            n324 = And(x=w705, y=w707) -> (x .and. y?=w703:bool)
            n325 = Not(x=w701) -> (.not. x?=w704:bool)
            n326 = And(x=w703, y=w704) -> (x .and. y?=w702:bool)
            n327 = case shown="True" w702 {
              frame False {
              }
              frame True {
                n328 = flat-sequence {
                  frame #0 {
                    w720 = TRUE
                    n329 = local read "TimeOutDuration"() -> (w721:i32)
                    n330 = xnode "DisplayOn 3"("C/DIO3 (DIO3)"=w720) -> ()  [unwired: 1 in, 1 out]
                    n331 = shared-variable "My Computer\\michelle_library.lvlib\\Timeout"(w720) -> ()  [unwired: 1 in, 1 out]
                    n332 = Wait (ms)(milliseconds to wait=w721) -> ()  [unwired: 1 out]
                    "Time_out" <- w720
                  }
                  frame #1 {
                    w757 = FALSE ("Timeout")
                    n333 = xnode "DisplayOn 4"("C/DIO3 (DIO3)"=w757) -> ()  [unwired: 1 in, 1 out]
                    n334 = local write "Time_out"(w757) -> ()
                    n335 = shared-variable "My Computer\\michelle_library.lvlib\\Timeout"(w757) -> ()  [unwired: 1 in, 1 out]
                  }
                }
              }
            }
            n336 = local read "Stop"() -> (w719:bool)
          }
          n337 = while {
            shift-right: [w870] -> _
            shift-left: _ -> [w869]
            shift-right: [w862] -> _
            shift-left: _ -> [w863]
            stop <- w872 stop-if-true
            n338 = local read "Active Trial"() -> (w867:bool)
            n339 = Wait (ms)(milliseconds to wait=u32 10) -> ()  [unwired: 1 out]
            n340 = local read "Lick"() -> (w868:bool)
            n341 = And(x=w867, y=w868) -> (x .and. y?=w866:bool)
            n342 = Or(x="Give reward", y=w866) -> (x .or. y?=w865:bool)
            n343 = case shown="True" w865 {
              tunnel: [w874 w881] -> w870
              tunnel: w869 -> [w874 w880]
              tunnel: w863 -> [w873 w878]
              tunnel: [w873 w877] -> w862
              frame False {
              }
              frame True {
                n344 = flat-sequence {
                  tunnel: w878 -> [w887]
                  tunnel: [w884] -> w875
                  tunnel: [w943] -> w876
                  tunnel: w875 -> [w941]
                  tunnel: [w987] -> w877
                  tunnel: w876 -> [w987]
                  frame #0 {
                    w902 = TRUE ("C/DIO0 (DIO0)")
                    n345 = Get Date/Time In Seconds() -> (seconds since 1Jan1904=w891:timestamp)
                    n346 = local write "Time_out"(FALSE) -> ()
                    n347 = shared-variable "My Computer\\michelle_library.lvlib\\Timeout"(FALSE) -> ()  [unwired: 1 in, 1 out]
                    n348 = local write "GoAhead"(FALSE) -> ()
                    n349 = Wait (ms)(milliseconds to wait=u32 100) -> ()  [unwired: 1 out]
                    n350 = local read "TestTime"() -> (w885:dbl)
                    n351 = shared-variable "My Computer\\michelle_library.lvlib\\Trial"() -> (w901:u32)  [unwired: 1 in, 1 out]
                    n352 = shared-variable "My Computer\\michelle_library.lvlib\\GlobalReward"() -> (w893:dbl)  [unwired: 1 in, 1 out]
                    n353 = To Double Precision Float(number=w891) -> (double precision float=w890:dbl)
                    n354 = shared-variable "My Computer\\michelle_library.lvlib\\GlobalTime"() -> (w883:dbl)  [unwired: 1 in, 1 out]
                    n355 = local read "Rewarded trials"() -> (w899:dbl[])
                    n356 = Subtract(x=w890, y=w885) -> (x-y=w889:dbl)
                    n357 = xnode "Reward 3"("C/DIO0 (DIO0)"=w902) -> ()  [unwired: 1 in, 1 out]
                    n358 = Decrement(x=w901) -> (x-1=w900:u32)
                    n359 = shared-variable "My Computer\\michelle_library.lvlib\\Frame_clock"() -> (w882:u32)  [unwired: 1 in, 1 out]
                    n360 = Increment(x=w893) -> (x+1=w892:dbl)
                    n361 = Replace Array Subset(array=w899, new element=1.0 ("new element/subarray"), index=w900) -> (w897:dbl[])
                    n362 = Build Array(551, w889, w883, w882) -> (w888:T1)
                    n363 = local write "Rewarded trials"(w897) -> ()
                    n364 = shared-variable "My Computer\\michelle_library.lvlib\\GlobalReward"(w892) -> ()  [unwired: 1 in, 1 out]
                    n365 = Build Array (concatenate) ("Build Matrix")(w887, w888) -> (w884:T1)
                    n366 = local write "RewTS"(w884) -> ()
                    "Reward" <- w902
                    "Watch_Display" <- w902
                  }
                  frame #1 {
                    w951 = FALSE ("C/DIO0 (DIO0)")
                    n367 = Get Date/Time In Seconds() -> (seconds since 1Jan1904=w948:timestamp)
                    n368 = local read "TestTime"() -> (w942:dbl)
                    n369 = local write "Give reward"(FALSE ("Give reward")) -> ()
                    n370 = Wait (ms)(milliseconds to wait=u32 20) -> ()  [unwired: 1 out]
                    n371 = shared-variable "My Computer\\michelle_library.lvlib\\GlobalTime"() -> (w940:dbl)  [unwired: 1 in, 1 out]
                    n372 = To Double Precision Float(number=w948) -> (double precision float=w947:dbl)
                    n373 = xnode "Reward 4"("C/DIO0 (DIO0)"=w951) -> ()  [unwired: 1 in, 1 out]
                    n374 = local write "Reward"(w951) -> ()
                    n375 = Subtract(x=w947, y=w942) -> (x-y=w946:dbl)
                    n376 = shared-variable "My Computer\\michelle_library.lvlib\\Frame_clock"() -> (w939:u32)  [unwired: 1 in, 1 out]
                    n377 = Build Array(552, w946, w940, w939) -> (w944:T1)
                    n378 = Build Array (concatenate) ("Build Matrix")(w941, w944) -> (w943:T1)
                    n379 = local write "RewTS"(w943) -> ()
                  }
                  frame #2 {
                    n380 = Wait (ms)(milliseconds to wait=u32 50) -> ()  [unwired: 1 out]
                  }
                }
                n381 = Increment(x=w880) -> (x+1=w881:u16)
                "Rewards" <- w881
                n382 = local write "Active Trial"(FALSE ("Active Trial")) -> ()
              }
            }
            n383 = local read "Stop"() -> (w872:bool)
          }
          n384 = while {
            stop <- w837 stop-if-true
            n385 = shared-variable "My Computer\\michelle_library.lvlib\\Trial"() -> (w833:u32)  [unwired: 1 in, 1 out]
            n386 = shared-variable "My Computer\\michelle_library.lvlib\\Trial"() -> (w829:u32)  [unwired: 1 in, 1 out]
            n387 = Wait (ms)(milliseconds to wait=u32 10) -> ()  [unwired: 1 out]
            n388 = local read "Rewarded trials"() -> (w830:dbl[])
            n389 = local read "Reward_mat"() -> (w832:dbl[])
            n390 = Decrement(x=w833) -> (x-1=w834:u32)
            n391 = Decrement(x=w829) -> (x-1=w828:u32)
            n392 = Index Array(array=w832, index=w834) -> (element=w835:dbl)
            n393 = Index Array(array=w830, index=w828) -> (element=w827:dbl)
            n394 = Equal To 0?(x=w827) -> (x = 0?=w826:bool)
            n395 = Equal?(x=w835, y=1.0) -> (x = y?=w825:bool)
            n396 = And(x=w825, y=w826) -> (x .and. y?=w824:bool)
            n397 = case shown="True" w824 {
              frame False {
                n398 = local write "Active Trial"(FALSE ("Active_trial")) -> ()
              }
              frame True {
                n399 = shared-variable "My Computer\\michelle_library.lvlib\\Trial"() -> (w840:u32)  [unwired: 1 in, 1 out]
                n400 = local read "Stim_ID"() -> (w842:dbl[])
                n401 = Decrement(x=w840) -> (x-1=w841:u32)
                n402 = Index Array(array=w842, index=w841) -> (element=w839:dbl)
                n403 = case shown="1, Default" w839 {
                  frame 1, Default {
                    n404 = shared-variable "My Computer\\michelle_library.lvlib\\ISI_Time"() -> (w848:dbl)  [unwired: 1 in, 1 out]
                    n405 = local read "ActiveTime"() -> (w843:dbl)
                    n406 = Less?(x=w848, y=w843) -> (x < y?=w846:bool)
                    n407 = Greater?(x=w848, y=0.1) -> (0:w845:bool)
                    n408 = And(x=w846, y=w845) -> (x .and. y?=w844:bool)
                    n409 = case shown="True" w844 {
                      frame False {
                        n410 = local write "Active Trial"(FALSE ("Active Trial")) -> ()
                      }
                      frame True {
                        n411 = local read "Time"() -> (w852:dbl)
                        n412 = local write "Active Trial"(TRUE ("Active Trial")) -> ()
                        n413 = Add(x=w852, y=-0.11) -> (x+y=w850:dbl)
                        n414 = local write "Time of last lick"(w850) -> ()
                      }
                    }
                  }
                  frame 2 {
                    n415 = shared-variable "My Computer\\michelle_library.lvlib\\ISI_Time"() -> (w858:dbl)  [unwired: 1 in, 1 out]
                    n416 = local read "ActiveTime"() -> (w854:dbl)
                    n417 = Less?(x=w858, y=w854) -> (x < y?=w856:bool)
                    n418 = Greater?(x=w858, y=0.1) -> (0:w857:bool)
                    n419 = And(x=w857, y=w856) -> (x .and. y?=w855:bool)
                    n420 = case shown="True" w855 {
                      frame False {
                        n421 = local write "Active Trial"(FALSE ("Active Trial")) -> ()
                      }
                      frame True {
                        "Active Trial" <- TRUE ("Active Trial")
                      }
                    }
                  }
                }
              }
            }
            n422 = local read "Stop"() -> (w837:bool)
          }
        }
      }
      n423 = flat-sequence {
        frame #0 {
          n424 = xnode "Encoder 4"("Reset Counter"=TRUE) -> ()  [unwired: 1 in, 4 out]
        }
        frame #1 {
          n425 = while {
            shift-right: [w393] -> _
            shift-left: _ -> [w394]
            stop <- w398 stop-if-true
            n426 = local read "GetVidFrame"() -> (w388:i32)
            n427 = local read "VidFrameClock"() -> (w392:i32)
            n428 = Equal?(x=w392, y=1) -> (x = y?=w391:bool)
            n429 = Equal?(x=w388, y=1) -> (x = y?=w387:bool)
            n430 = And(x=w391, y=w387) -> (x .and. y?=w390:bool)
            n431 = case shown="True" w390 {
              tunnel: w394 -> [w402 w405]
              tunnel: [w402 w404] -> w393
              frame False {
              }
              frame True {
                n432 = local read "TestTime"() -> (w411:dbl)
                n433 = shared-variable "My Computer\\michelle_library.lvlib\\GlobalTime"() -> (w408:dbl)  [unwired: 1 in, 1 out]
                n434 = Get Date/Time In Seconds() -> (seconds since 1Jan1904=w413:timestamp)
                n435 = shared-variable "My Computer\\michelle_library.lvlib\\Frame_clock"() -> (w409:u32)  [unwired: 1 in, 1 out]
                n436 = To Double Precision Float(number=w413) -> (double precision float=w412:dbl)
                n437 = Subtract(x=w412, y=w411) -> (x-y=w410:dbl)
                n438 = Build Array(881, w410, w408, w409) -> (w407:T1)
                n439 = Build Array (concatenate) ("Build Matrix")(w405, w407) -> (w404:T1)
                n440 = local write "GetVidFrame"(0) -> ()
                n441 = local write "VidTS"(w404) -> ()
              }
            }
            n442 = xnode "Encoder 3"() -> ("Counter Value"=w400:i32)  [unwired: 2 in, 3 out]
            n443 = Multiply(x=w400, y=-1) -> (x*y=w397:i32)
            "VidFrameClock" <- w397
            n444 = Equal?(x=w397, y=720000) -> (x = y?=w398:bool)
            n445 = shared-variable "My Computer\\michelle_library.lvlib\\VidFrameClock1"(w397) -> ()  [unwired: 1 in, 1 out]
            n446 = local write "Stop"(w398) -> ()
            n447 = Wait (ms)(milliseconds to wait=u32 1) -> ()  [unwired: 1 out]
          }
        }
        frame #2 {
          n448 = local read "Stop"() -> (w460:bool)
          n449 = shared-variable "My Computer\\michelle_library.lvlib\\Stop"(w460) -> ()  [unwired: 1 in, 1 out]
        }
      }
    }
  }
